vi "MSGR Receive (Refnum).vi"(0 "MSGR Q":refnum<queue>, 11 "error in (no error)":errorcluster, 12 "timeout in ms (-1)":i32=-1) -> (6 "MSGR Q Data TypeDef":T1, 14 "timed out?":bool, 15 "error out":errorcluster)   [LabVIEW 2018]
doc: "MIT License\n\nCopyright (c) 2020 RichardLGP5\n\nPermission is hereby granted, free of charge, to any person obtaining a copy\nof this software and associated documentation files (the \"Software\"), to deal\nin the Software without restriction, including without limitation the rights\nto use, copy, modify, merge, publish, distribute, sublicense, and/or sell\ncopies of the Software, and to permit persons to whom the Software is\nfurnished to do so, subject to the following conditions:\n\nThe above copyright notice and this permission notice shall be included in all\ncopies or substantial portions of the Software.\n\nTHE SOFTWARE IS PROVIDED \"AS IS\", WITHOUT WARRANTY OF ANY KIND, EXPRESS OR\nIMPLIED, INCLUDING BUT NOT LIMITED TO THE WARRANTIES OF MERCHANTABILITY,\nFITNESS FOR A PARTICULAR PURPOSE AND NONINFRINGEMENT. IN NO EVENT SHALL THE\nAUTHORS OR COPYRIGHT HOLDERS BE LIABLE FOR ANY CLAIM, DAMAGES OR OTHER\nLIABILITY, WHETHER IN AN ACTION OF CONTRACT, TORT OR OTHERWISE, ARISING FROM,\nOUT OF OR IN CONNECTION WITH THE SOFTWARE OR THE USE OR OTHER DEALINGS IN THE\nSOFTWARE."
uses:
  MSGR Q Data TypeDef.ctl
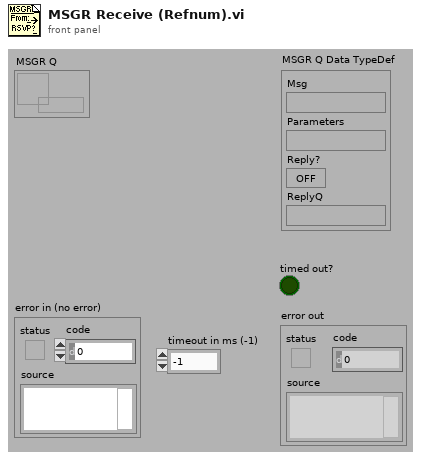
[diagram p1: front panel]
types:
  T1 = typedef "MSGR Q Data TypeDef.ctl" = cluster{"Msg":string, "Parameters":string, "Reply?":bool, "ReplyQ":string}
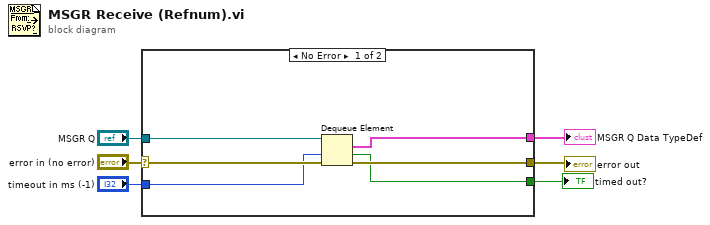
[diagram p0: block diagram]
diagram:
  n1 = case shown="No Error" "error in (no error)" {
    selector: "error in (no error)" -> [w10 w13]
    tunnel: [w12 w13] -> w6
    tunnel: "MSGR Q" -> [w11 _]
    tunnel: [w7 _] -> w3
    tunnel: [w9 _] -> w2
    tunnel: "timeout in ms (-1)" -> [w8 _]
    frame No Error {
      n2 = Dequeue Element(queue=w11, timeout in ms (-1)=w8, error in (no error)=w10) -> (element=w7:T1, timed out?=w9:bool, error out=w12:errorcluster)  [unwired: 1 out]
    }
    frame Error {
    }
  }
  "error out" <- w6
  "MSGR Q Data TypeDef" <- w3
  "timed out?" <- w2
